vi "cuadrado magico.vi"() -> ()   [LabVIEW 2021]
panel:
  out "indicador index":i32
  in  "bandera":i32
  in  "j_anterior":i32=2
  in  "i_anterior":i32
  in  "index":i32
  in  "tem":i32=1
  in  "j":i32=2
  in  "i":i32
  out "Array":i32[][](array[numeric])=[[15, 17, 18], [20, 21, 23], [24, 26, 27]]
  in  "punto_incial":i32=2
  out "warring":string="ok"
  in  "Orden de la matriz":i32=3
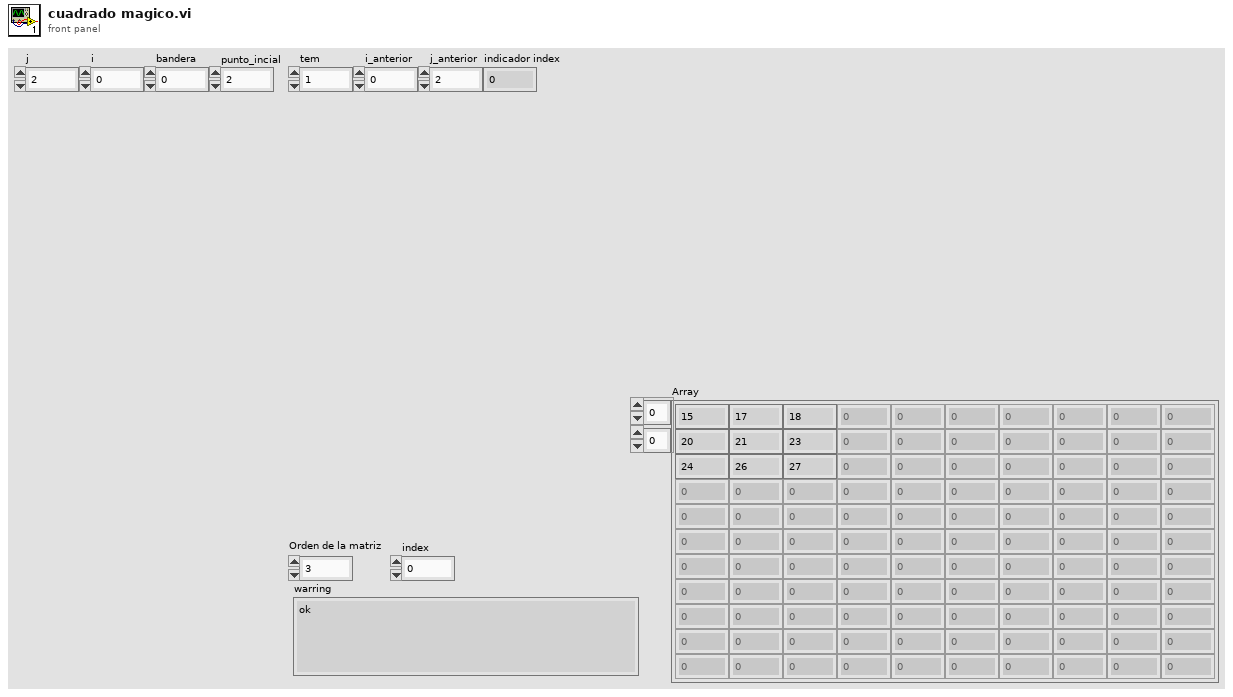
[diagram p1: front panel]
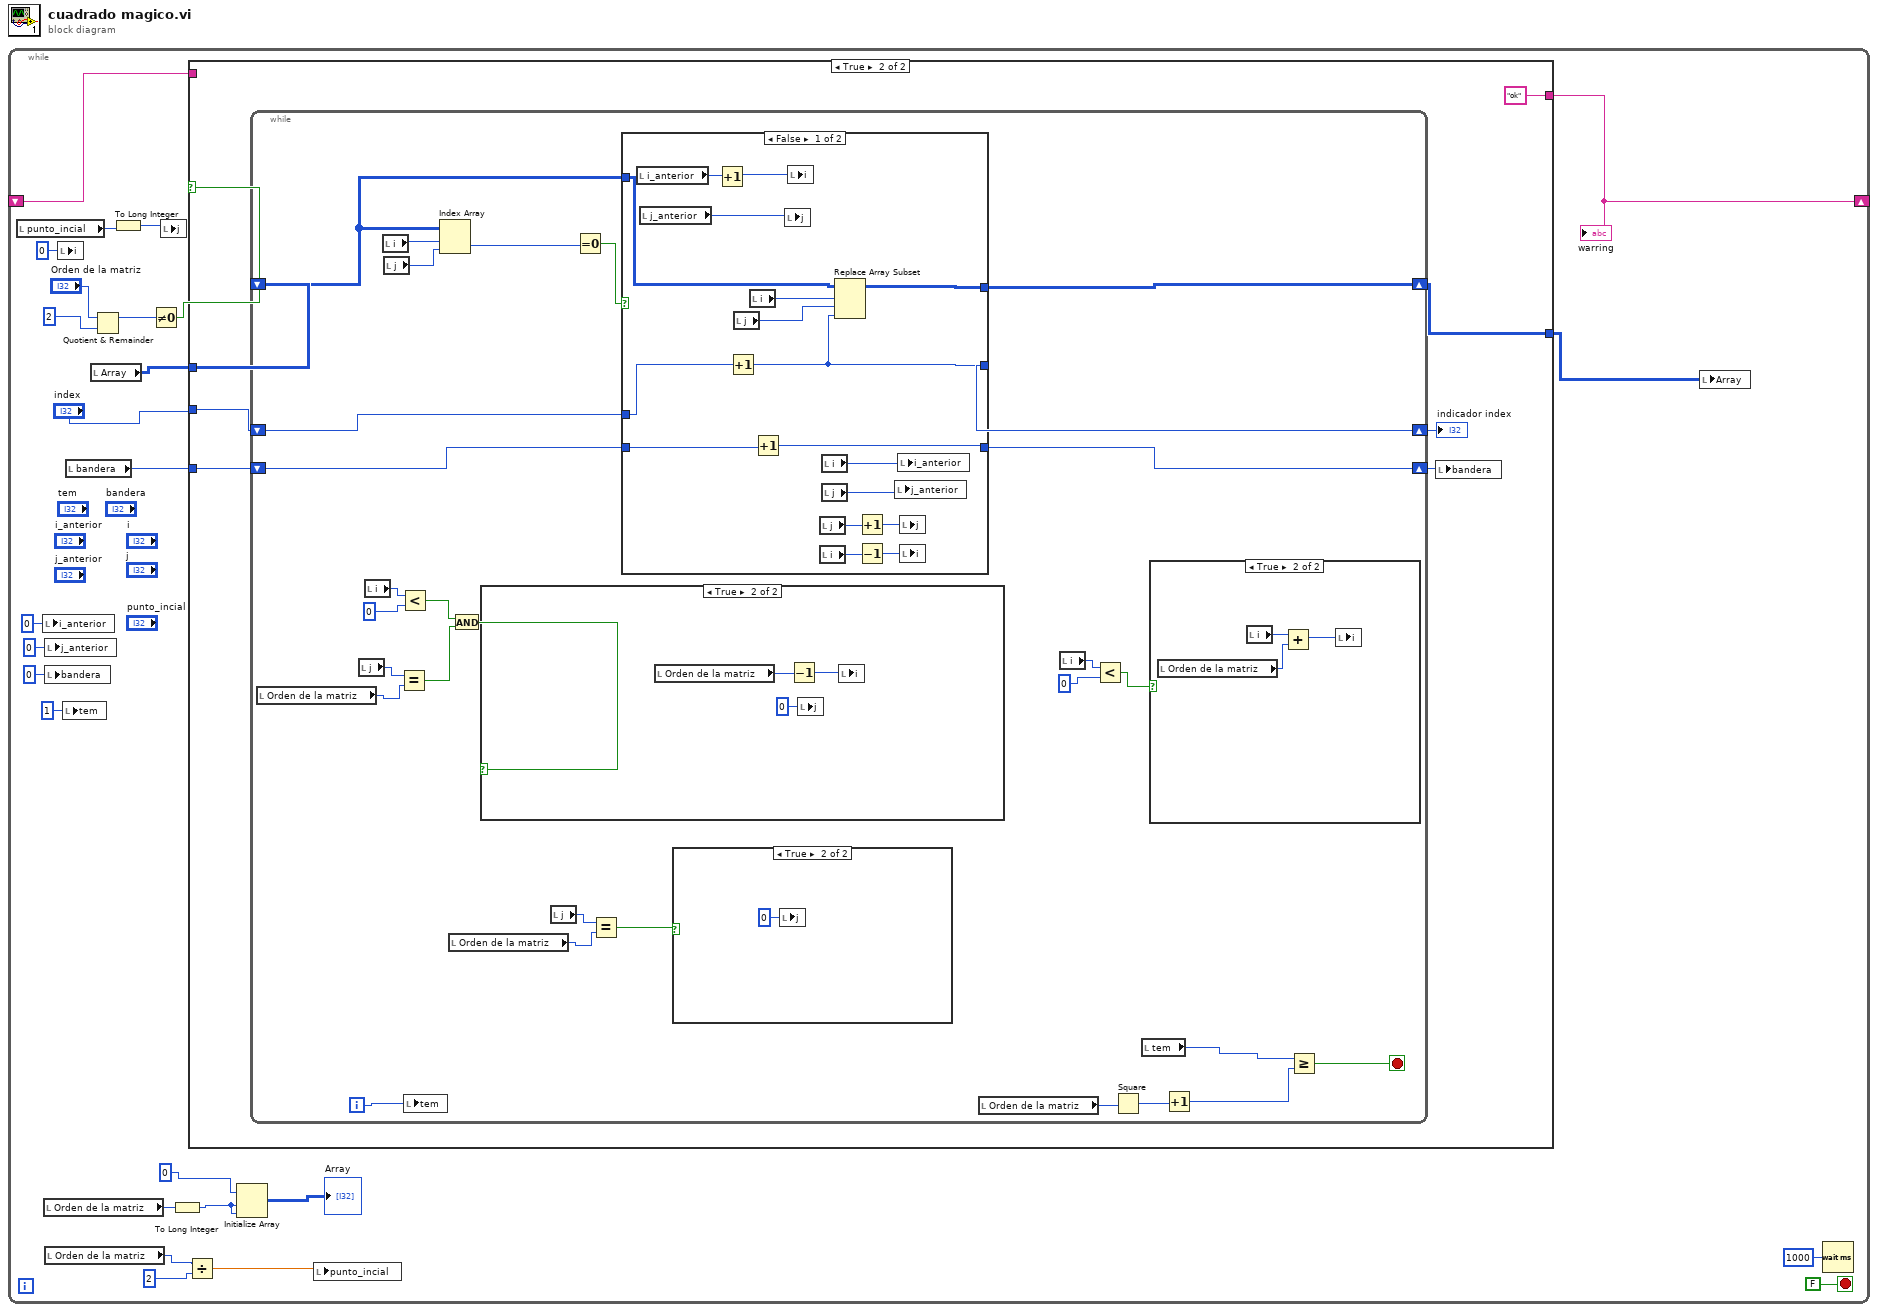
[diagram p0: block diagram]
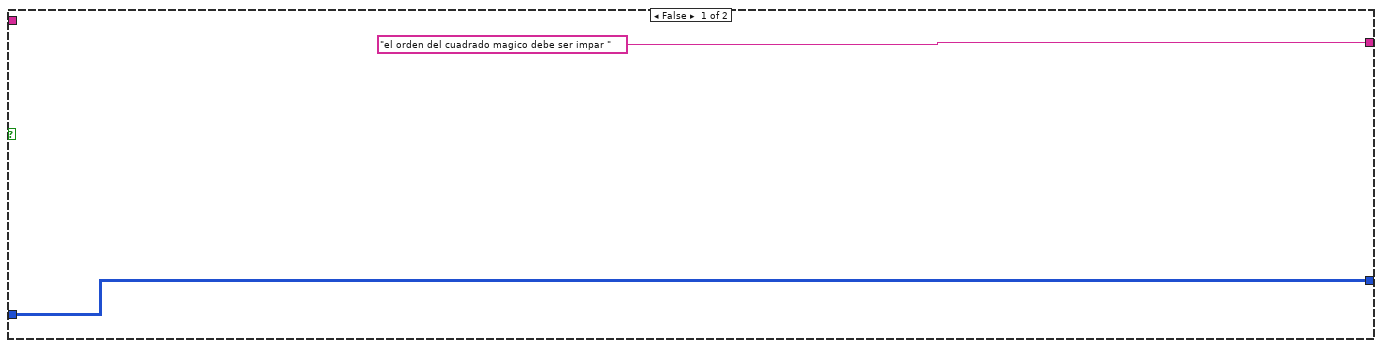
[diagram p2: hidden frame]
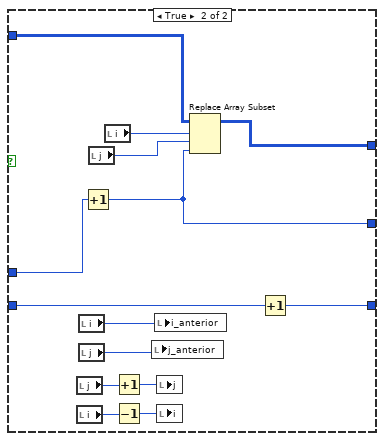
[diagram p6: hidden frame]
diagram:
  n1 = while {
    shift-right: [w24] -> _
    shift-left: _ -> [w25]
    stop <- FALSE stop-if-true
    n2 = local read "punto_incial"() -> (w15:i32)
    n3 = local write "i_anterior"(0 ("i_anterior")) -> ()
    n4 = local read "Orden de la matriz"() -> (w9:i32)
    n5 = local write "j_anterior"(0 ("j_anterior")) -> ()
    n6 = local write "bandera"(0 ("bandera")) -> ()
    n7 = local read "Orden de la matriz"() -> (w6:i32)
    n8 = local write "i"(0 ("i")) -> ()
    n9 = local write "tem"(1 ("tem")) -> ()
    n10 = local read "bandera"() -> (w11:i32)
    n11 = local read "Array"() -> (w13:i32[][])
    n12 = Quotient & Remainder(x="Orden de la matriz", y=2) -> (x-y*floor(x/y)=w20:i32)  [unwired: 1 out]
    n13 = To Long Integer(number=w15) -> (32bit integer=w14:i32)
    n14 = Not Equal To 0?(x=w20) -> (x != 0?=w21:bool)
    n15 = local write "j"(w14) -> ()
    n16 = To Long Integer(number=w9) -> (32bit integer=w8:i32)
    n17 = Divide(x=w6, y=2) -> (x/y=w4:dbl)
    n18 = case shown="True" w21 {
      tunnel: ["el orden del cuadrado magico debe ser impar " "ok"] -> w24
      tunnel: w25 -> [_ _]
      tunnel: w13 -> [w27 w34]
      tunnel: [w27 w33] -> w1
      tunnel: w11 -> [_ w32]
      tunnel: "index" -> [_ w29]
      frame False {
      }
      frame True {
        n19 = while {
          shift-right: [w54] -> w33
          shift-left: w34 -> [w58]
          shift-right: [w52] -> w31
          shift-left: w32 -> [w53]
          shift-right: [w51] -> w30
          shift-left: w29 -> [w56]
          i -> [w55]
          stop <- w61 stop-if-true
          n20 = local read "Orden de la matriz"() -> (w45:i32)
          n21 = local read "j"() -> (w46:i32)
          n22 = local read "i"() -> (w49:i32)
          n23 = local read "i"() -> (w57:i32)
          n24 = local read "j"() -> (w36:i32)
          n25 = Equal?(x=w46, y=w45) -> (x = y?=w44:bool)
          n26 = Less?(x=w49, y=0) -> (x < y?=w47:bool)
          n27 = local write "tem"(w55) -> ()
          n28 = Index Array(array=w58, index (row)=w57, index (col)=w36) -> (element=w60:i32)
          n29 = local read "Orden de la matriz"() -> (w37:i32)
          n30 = And(x=w47, y=w44) -> (x .and. y?=w43:bool)
          n31 = case shown="True" w43 {
            frame False {
            }
            frame True {
              n32 = local read "Orden de la matriz"() -> (w71:i32)
              n33 = Decrement(x=w71) -> (x-1=w70:i32)
              n34 = local write "j"(0 ("j")) -> ()
              n35 = local write "i"(w70) -> ()
            }
          }
          n36 = local read "j"() -> (w38:i32)
          n37 = Equal To 0?(x=w60) -> (x = 0?=w59:bool)
          n38 = Equal?(x=w38, y=w37) -> (x = y?=w39:bool)
          n39 = case shown="False" w59 {
            tunnel: w58 -> [w82 w100]
            tunnel: [w81 w99] -> w54
            tunnel: w56 -> [w83 w98]
            tunnel: [w80 w97] -> w51
            tunnel: [w78 w96] -> w52
            tunnel: w53 -> [w79 w95]
            frame False {
              n40 = local read "i_anterior"() -> (w87:i32)
              n41 = local read "j_anterior"() -> (w86:i32)
              n42 = Increment(x=w87) -> (x+1=w88:i32)
              n43 = Increment(x=w83) -> (x+1=w80:i32)
              n44 = local read "j"() -> (w84:i32)
              n45 = local read "i"() -> (w85:i32)
              n46 = Increment(x=w79) -> (x+1=w78:i32)
              n47 = local write "j"(w86) -> ()
              n48 = local write "i"(w88) -> ()
              n49 = local read "j"() -> (w74:i32)
              n50 = local read "i"() -> (w76:i32)
              n51 = local read "i"() -> (w72:i32)
              n52 = local read "j"() -> (w73:i32)
              n53 = Replace Array Subset(array=w82, new element=w80, index (row)=w85, index (col)=w84) -> (w81:i32[][])
              n54 = Increment(x=w74) -> (x+1=w75:i32)
              n55 = Decrement(x=w76) -> (x-1=w77:i32)
              n56 = local write "j_anterior"(w73) -> ()
              n57 = local write "i_anterior"(w72) -> ()
              n58 = local write "j"(w75) -> ()
              n59 = local write "i"(w77) -> ()
            }
            frame True {
              n60 = local read "j"() -> (w91:i32)
              n61 = local read "i"() -> (w93:i32)
              n62 = local read "i"() -> (w89:i32)
              n63 = local read "j"() -> (w90:i32)
              n64 = Increment(x=w98) -> (x+1=w97:i32)
              n65 = local read "j"() -> (w101:i32)
              n66 = local read "i"() -> (w102:i32)
              n67 = Increment(x=w91) -> (x+1=w92:i32)
              n68 = Decrement(x=w93) -> (x-1=w94:i32)
              n69 = local write "j_anterior"(w90) -> ()
              n70 = local write "i_anterior"(w89) -> ()
              n71 = local write "j"(w92) -> ()
              n72 = local write "i"(w94) -> ()
              n73 = Replace Array Subset(array=w100, new element=w97, index (row)=w102, index (col)=w101) -> (w99:i32[][])
              n74 = Increment(x=w95) -> (x+1=w96:i32)
            }
          }
          n75 = case shown="True" w39 {
            frame False {
            }
            frame True {
              n76 = local write "j"(0 ("j")) -> ()
            }
          }
          n77 = local read "Orden de la matriz"() -> (w64:i32)
          n78 = local read "i"() -> (w41:i32)
          n79 = Less?(x=w41, y=0) -> (x < y?=w42:bool)
          n80 = Square(x=w64) -> (x^2=w63:i32)
          n81 = local read "tem"() -> (w50:i32)
          n82 = case shown="True" w42 {
            frame False {
            }
            frame True {
              n83 = local read "Orden de la matriz"() -> (w67:i32)
              n84 = local read "i"() -> (w68:i32)
              n85 = Add(x=w68, y=w67) -> (x+y=w66:i32)
              n86 = local write "i"(w66) -> ()
            }
          }
          n87 = Increment(x=w63) -> (x+1=w62:i32)
          n88 = Greater Or Equal?(x=w50, y=w62) -> (x >= y?=w61:bool)
        }
        "indicador index" <- w30
        n89 = local write "bandera"(w31) -> ()
      }
    }
    "warring" <- w24
    n90 = Initialize Array "Initialize Array"(0, w8, w8) -> (→"Array":i32[][])
    n91 = local write "punto_incial"(w4) -> ()
    n92 = local write "Array"(w1) -> ()
    n93 = Wait (ms)(milliseconds to wait=u32 1000) -> ()  [unwired: 1 out]
  }
